vi "GetJSONData.vi"(0 "reference in":refnum<class "String.lvclass">, 2 "VI Reference":refnum<vi>, 5 "error in (no error)":errorcluster) -> (14 "reference out":refnum<class "String.lvclass">, 15 "JSON string":string, 19 "error out":errorcluster)   [LabVIEW 2014, in "FrontPanelPublisher.lvlib" / "String.lvclass"]
uses:
  String.lvclass
  Control_class/Control.lvclass
  Object_class/Object.lvclass
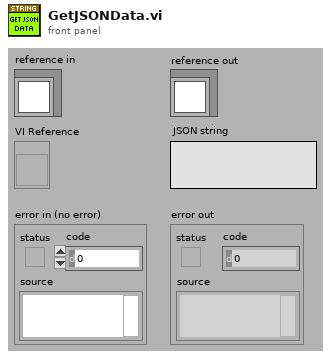
[diagram p1: front panel]
types:
  T1 = typedef "FrontPanelPublisher.lvlib/Object.lvclass/Attributes.ctl" = cluster{"UID":i32, "Type":string, "Coordinates":T2, "Reference":refnum<vi>}
  T2 = typedef "FrontPanelPublisher.lvlib/Object.lvclass/Coordinates.ctl" = cluster{"Left":i32, "Top":i32, "Height":u32, "Width":u32}
  T3 = typedef "FrontPanelPublisher.lvlib/Control.lvclass/Attributes.ctl" = cluster{"Description":string, "Indicator":bool, "Default Value":variant, "Control Index":i32, "Label":refnum<class "Text.lvclass">, "Caption":refnum<class "Text.lvclass">, "Use Picture":bool, "Image1 b64":string, "Image2 b64":string}
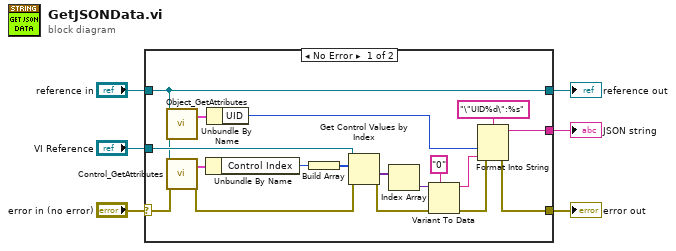
[diagram p0: block diagram]
diagram:
  n1 = case shown="No Error" "error in (no error)" {
    selector: "error in (no error)" -> [w24 w26]
    tunnel: [w20 w26] -> w5
    tunnel: [w9 w25] -> w3
    tunnel: "reference in" -> [w9 w25]
    tunnel: "VI Reference" -> [w14 _]
    tunnel: [w10 _] -> w1
    frame No Error {
      n2 = call "Object_GetAttributes.vi"("reference in"=w9) -> ("Data"=w8:T1)  [unwired: 15 in, 3 out]
      n3 = call "Control_GetAttributes.vi"("reference in"=w9, "error in (no error)"=w24) -> ("Data"=w19:T3, "error out"=w21:errorcluster)  [unwired: 14 in, 2 out]
      n4 = Unbundle By Name(w19) -> ("Control Index"=w18:i32)
      n5 = Unbundle By Name(w8) -> ("UID"=w7:i32)
      n6 = Build Array(w18) -> (w17:i32[])
      n7 = Get Control Values by Index(0:w14, 1:w17, 3:w21) -> (10:w15:variant[], 11:w23:errorcluster)
      n8 = Index Array(array=w15) -> (element=w13:variant)  [unwired: 1 in]
      n9 = Variant To Data(error in=w23, type="0", Variant=w13) -> (data=w11:string, error out=w22:errorcluster)
      n10 = Format Into String(format string="\"UID%d\":%s", error in=w22, w7, w11) -> (resulting string=w10:string, error out=w20:errorcluster)  [unwired: 1 in]
    }
    frame Error {
    }
  }
  "error out" <- w5
  "reference out" <- w3
  "JSON string" <- w1
